vi "White Noise adder - robots.vi"(9 "robots":T1[](array[typedef]) {"height" format="%+4.3f"; "pixel_y" format="%+4.3f"; "pixel_x" format="%+4.3f"; "orientation" format="%+4.3f"; "y" format="%+4.3f"; "confidence" format="%4.3f"; "x" format="%+4.3f"}) -> (3 "Robots w noise":T1[](array[typedef]) {"height" format="%+4.3f"; "pixel_y" format="%+4.3f"; "pixel_x" format="%+4.3f"; "orientation" format="%+4.3f"; "y" format="%+4.3f"; "confidence" format="%4.3f"; "x" format="%+4.3f"})   [LabVIEW 2016]
uses:
  SSL Detection Robot.ctl
  <vilib>/Analysis/NI_AALBase.lvlib
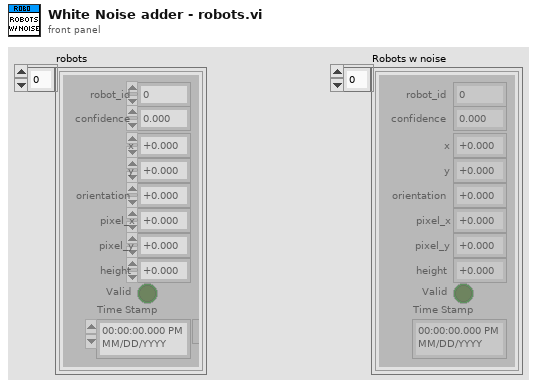
[diagram p1: front panel]
types:
  T1 = typedef "SSL Detection Robot.ctl" = cluster{"x":sgl, "robot_id":u32, "confidence":sgl, "y":sgl, "orientation":sgl, "pixel_x":sgl, "pixel_y":sgl, "height":sgl, "Valid":bool, "Time Stamp":timestamp}
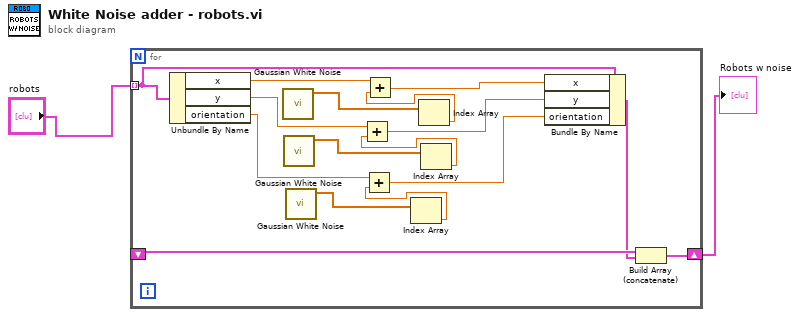
[diagram p0: block diagram]
diagram:
  n1 = for {
    tunnel: "robots" -> [w18] mode=indexing
    shift-right: [w5] -> w1
    shift-left: _ -> [w4]
    n2 = Unbundle By Name(w18) -> ("x"=w15:sgl, "y"=w16:sgl, "orientation"=w17:sgl)
    n3 = call <vilib>:"Gaussian White Noise.vi"() -> ("Gaussian noise pattern"=w14:dbl[])  [unwired: 10 in, 1 out]
    n4 = call <vilib>:"Gaussian White Noise.vi"() -> ("Gaussian noise pattern"=w11:dbl[])  [unwired: 10 in, 1 out]
    n5 = call <vilib>:"Gaussian White Noise.vi"() -> ("Gaussian noise pattern"=w8:dbl[])  [unwired: 10 in, 1 out]
    n6 = Index Array(array=w8) -> (element=w7:dbl)  [unwired: 1 in]
    n7 = Add(x=w17, y=w7) -> (x+y=w6:dbl)
    n8 = Index Array(array=w14) -> (element=w13:dbl)  [unwired: 1 in]
    n9 = Add(x=w15, y=w13) -> (x+y=w12:dbl)
    n10 = Index Array(array=w11) -> (element=w10:dbl)  [unwired: 1 in]
    n11 = Add(x=w16, y=w10) -> (x+y=w9:dbl)
    n12 = Bundle By Name(cluster=w18, "x"=w12, "y"=w9, "orientation"=w6) -> (w3:T1)
    n13 = Build Array (concatenate)(w4, w3) -> (w5:T1[])
  }
  "Robots w noise" <- w1
